vi "车牌识别模块.vi"(11 "图片路径":string="E:\\Program Files (x86)\\National Instruments\\LabVIEW 2013\\data\\记录照片\\00_20160426_110007.bmp") -> (0 "识别结果":T1, 3 "识别成功？":bool, 4 "加密狗插入？":bool)   [LabVIEW 2013]
uses:
  <vilib>/Utility/importsl/GetValueByPointer/datatype.ctl
  <vilib>/Utility/importsl/GetValueByPointer/GetValueByPointer.xnode
panel:
  out "pResult":string
  out "置信度":i32
  out "颜色":string
  out "车牌数目":i32
  out "左上Y":i32
  out "右下X":i32
  out "右下Y":i32
  out "左上X":i32
  out "车牌内容":string
  in  "HRIVLprOcx":refnum<k7>(container)
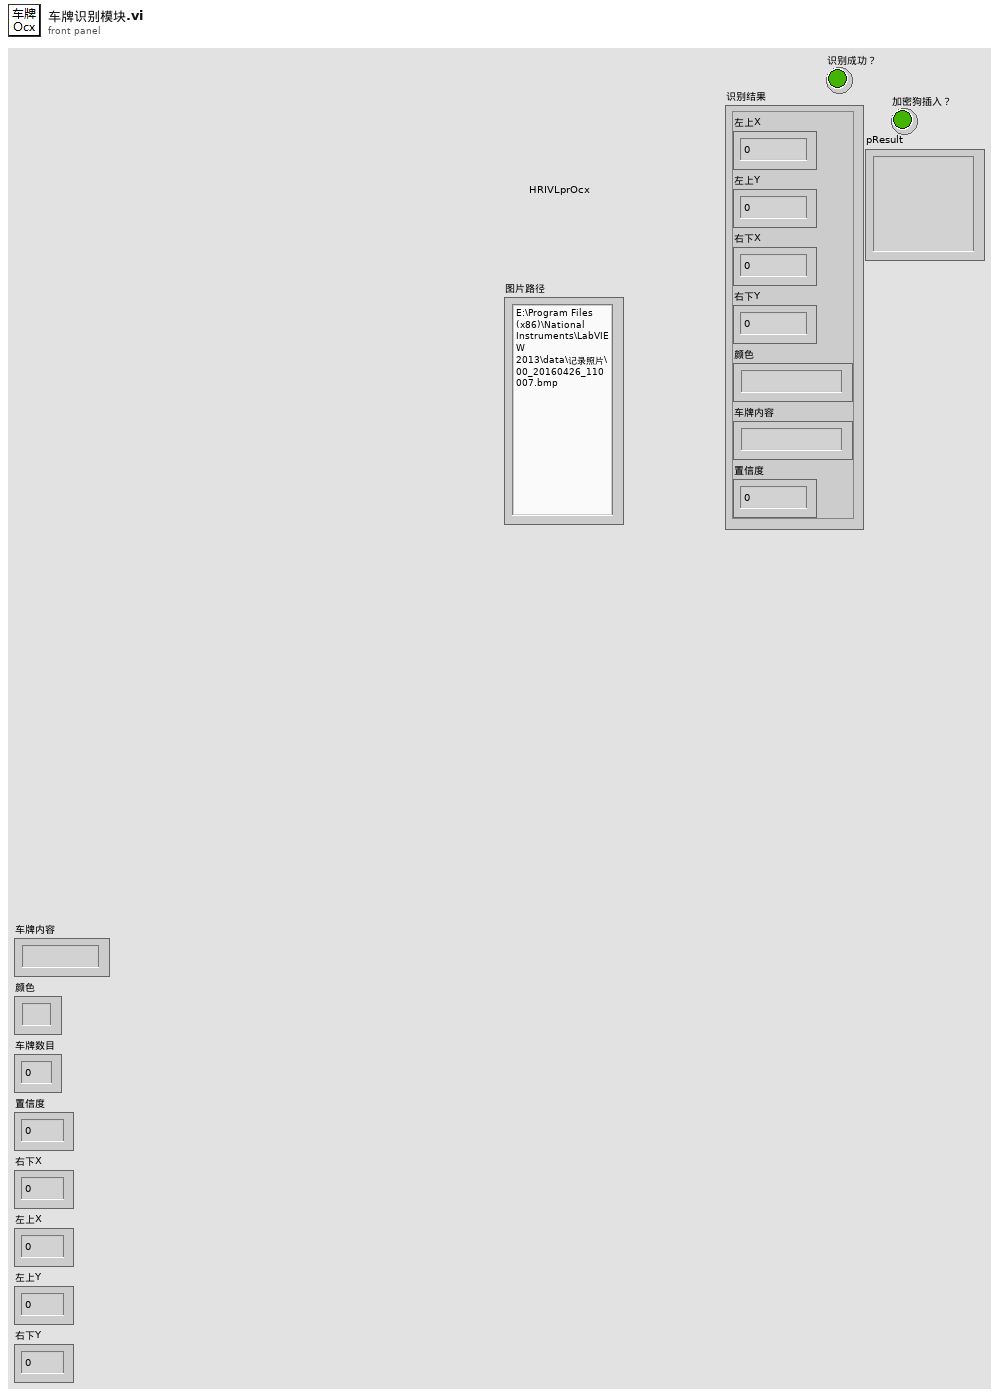
[diagram p1: front panel]
types:
  T1 = cluster{"左上X":i32, "左上Y":i32, "右下X":i32, "右下Y":i32, "颜色":string, "车牌内容":string, "置信度":i32}
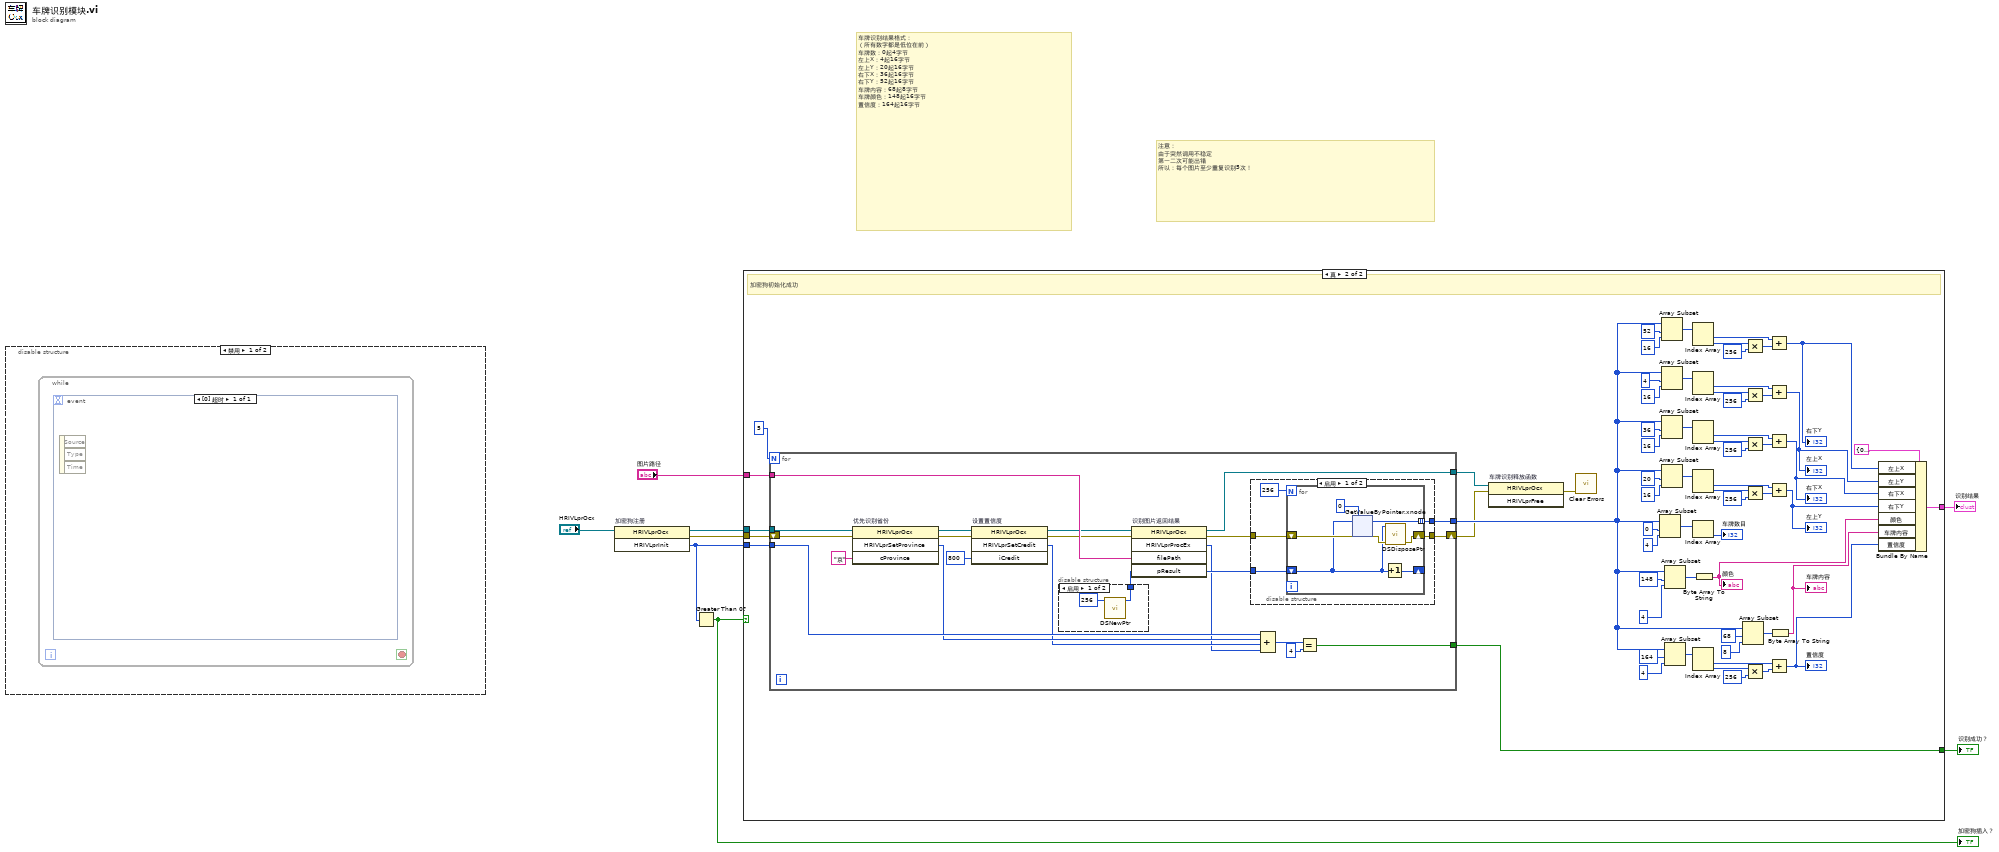
[diagram p0: block diagram]
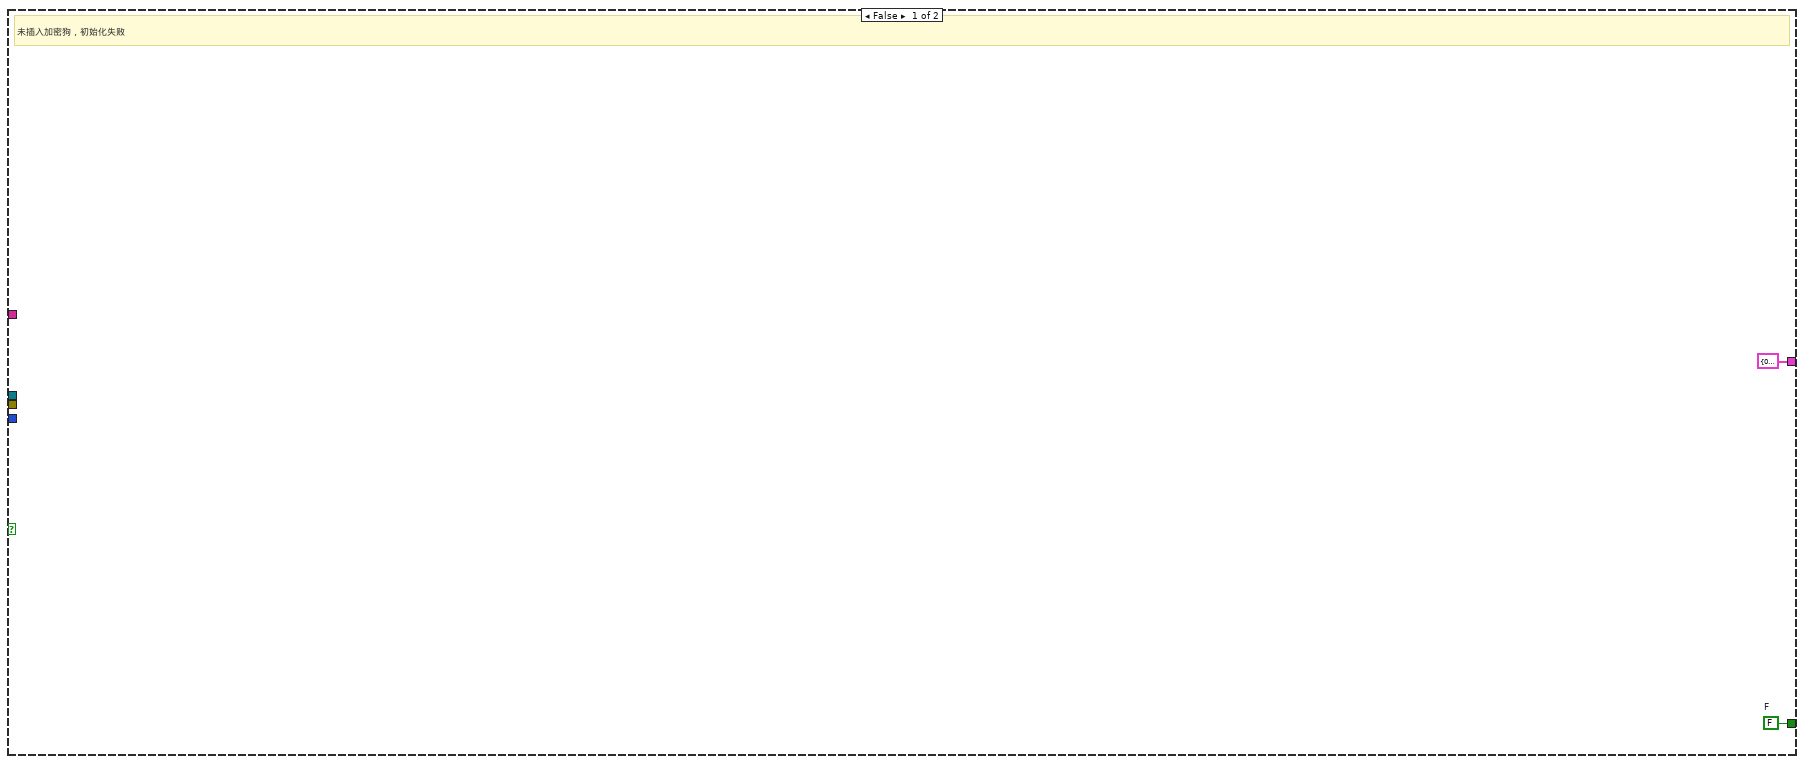
[diagram p3: hidden frame]
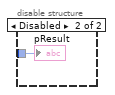
[diagram p5: hidden frame]
diagram:
  # "注意：\n由于突然调用不稳定\n第一二次可能出错\n所以：每个图片至少重复识别5次！"
  # "车牌识别结果格式：\n（所有数字都是低位在前）\n车牌数：0起4字节\n左上X：4起16字节\n左上Y：20起16字节\n右下X：36起16字节\n右下Y：52起16字节\n车牌内容：68起8字节\n车牌颜色：148起16字节\n置信度：164起16字节"
  n1 = disable-structure shown="禁用" {
    frame Disabled {
      n2 = while {
        stop <- _ stop-if-true
        n3 = event shown="[0] 超时" {
          selector: _ -> [_]
          dyn-events: _ -> [_]
          timeout: _ -> [_]
          event Timeout {
            n4 = event-data() -> ()  [unwired: 1 in, 3 out]
          }
        }
      }
    }
    frame Enabled {
    }
  }
  n5 = invoke on="加密狗注册" class="HRIVLprOcx" method="HRIVLprInit"(reference="HRIVLprOcx") -> (reference out=w7:refnum<k7>, error out=w4:errorcluster, "HRIVLprInit"=w1:i32)  [unwired: 2 in]
  n6 = Greater Than 0?(x=w1) -> (x > 0?=w2:bool)
  "加密狗插入？" <- w2
  n7 = case shown="真" w2 {
    tunnel: w7 -> [_ w74]
    tunnel: "图片路径" -> [_ w73]
    tunnel: w1 -> [_ w26]
    tunnel: [T1 {"左上X"=0, "左上Y"=0, "右下X"=0, "右下Y"=0, "颜色"="", "车牌内容"="", "置信度"=0} ("输出簇 2") w19] -> w5
    tunnel: w4 -> [_ w14]
    tunnel: [w10 w11] -> w3
    frame False {
      w10 = FALSE  # F
      # "未插入加密狗，初始化失败"
    }
    frame True {
      # "加密狗初始化成功"
      n8 = for {
        N: 5 -> [_]
        tunnel: w74 -> [w96]
        tunnel: w73 -> [w95]
        tunnel: [w94] -> w27
        tunnel: w26 -> [w93]
        tunnel: [w79] -> w15
        shift-right: [w78] -> w13
        shift-left: w14 -> [w77]
        tunnel: [w76] -> w11
        n9 = invoke on="优先识别省份" class="HRIVLprOcx" method="HRIVLprSetProvince"(reference=w96, error in=w77, "cProvince"="京") -> (reference out=w91:refnum<k7>, error out=w88:errorcluster, "HRIVLprSetProvince"=w85:i32)  [unwired: 1 in, 1 out]
        n10 = invoke on="设置置信度" class="HRIVLprOcx" method="HRIVLprSetCredit"(reference=w91, error in=w88, "iCredit"=800) -> (reference out=w89:refnum<k7>, error out=w87:errorcluster, "HRIVLprSetCredit"=w84:i32)  [unwired: 1 in, 1 out]
        n11 = disable-structure shown="启用" {
          disable-tunnel: [w97 _] -> w75
          frame Enabled {
            n12 = call <vilib>:"DSNewPtr.vi"("Size"=u64 256) -> ("Pointer"=w97:u64)  [unwired: 9 in, 1 out]
          }
          frame Disabled {
          }
        }
        n13 = invoke on="识别图片返回结果" class="HRIVLprOcx" method="HRIVLprProcEx"(reference=w89, error in=w87, "filePath"=w95, "pResult"=w75) -> (reference out=w79:refnum<k7>, error out=w80:errorcluster, "HRIVLprProcEx"=w83:i32, "pResult"=w86:i32)  [unwired: 1 in, 1 out]
        n14 = disable-structure shown="启用" {
          disable-tunnel: [w103 _] -> w94
          disable-tunnel: w86 -> [w101 w123]
          disable-tunnel: w80 -> [w100 _]
          disable-tunnel: [w99 _] -> w78
          frame Enabled {
            n15 = for {
              N: 256 -> [_]
              shift-right: [w110] -> _
              shift-left: w101 -> [w104]
              tunnel: [w108] -> w103 mode=indexing
              shift-right: [w105] -> w99
              shift-left: w100 -> [w107]
              n16 = xnode "GetValueByPointer.xnode"("Pointer"=w104, "InputType"=u8 0, "ErrorIn"=w107) -> ("Output"=w108:u8, "ErrorOut"=w106:errorcluster)  [unwired: 1 in]
              n17 = Increment(x=w104) -> (x+1=w110:i32)
              n18 = call <vilib>:"DSDisposePtr.vi"("error in (no error)"=w106, "Pointer"=w104) -> ("error out"=w105:errorcluster)  [unwired: 9 in]
            }
          }
          frame Disabled {
            "pResult" <- w123
          }
        }
        n19 = Compound Arithmetic op=ADD(w93, w85, w84, w83) -> (w82:i32)
        n20 = Equal?(x=w82, y=4) -> (x = y?=w76:bool)
      }
      n21 = invoke on="车牌识别释放函数" class="HRIVLprOcx" method="HRIVLprFree"(reference=w15, error in=w13) -> (error out=w12:errorcluster)  [unwired: 1 in, 2 out]
      n22 = call <vilib>:"Clear Errors.vi"("error in (no error)"=w12) -> ()  [unwired: 6 in, 1 out]
      n23 = Array Subset(array=w27, index=0 ("索引"), length=4 ("长度")) -> (w61:u8[])
      n24 = Array Subset(array=w27, index=52 ("索引"), length=16 ("长度")) -> (w60:u8[])
      n25 = Array Subset(array=w27, index=4 ("索引"), length=16 ("长度")) -> (w41:u8[])
      n26 = Array Subset(array=w27, index=36 ("索引"), length=16 ("长度")) -> (w59:u8[])
      n27 = Array Subset(array=w27, index=20 ("索引"), length=16 ("长度")) -> (w58:u8[])
      n28 = Array Subset(array=w27, index=148 ("索引"), length=4 ("长度")) -> (w65:u8[])
      n29 = Array Subset(array=w27, index=164 ("索引"), length=4 ("长度")) -> (w72:u8[])
      n30 = Index Array(array=w60) -> (element #1=w49:u8, element #2=w46:u8)  [unwired: 2 in]
      n31 = Index Array(array=w41) -> (element #1=w42:u8, element #2=w45:u8)  [unwired: 2 in]
      n32 = Index Array(array=w59) -> (element #1=w50:u8, element #2=w53:u8)  [unwired: 2 in]
      n33 = Index Array(array=w58) -> (element #1=w57:u8, element #2=w54:u8)  [unwired: 2 in]
      n34 = Index Array(array=w61) -> (element=→"车牌数目":u8)  [unwired: 1 in]
      n35 = Index Array(array=w72) -> (element #1=w68:u8, element #2=w71:u8)  [unwired: 2 in]
      n36 = Byte Array To String(unsigned byte array=w65) -> (string=w21:string)
      "颜色" <- w21
      n37 = Array Subset(array=w27, index=68 ("索引"), length=8 ("长度")) -> (w32:u8[])
      n38 = Multiply(x=w46, y=256) -> (x*y=w48:i32)
      n39 = Multiply(x=w45, y=256) -> (x*y=w43:i32)
      n40 = Multiply(x=w53, y=256) -> (x*y=w51:i32)
      n41 = Multiply(x=w54, y=256) -> (x*y=w56:i32)
      n42 = Multiply(x=w71, y=256) -> (x*y=w69:i32)
      n43 = Add(x=w49, y=w48) -> (x+y=w25:i32)
      "右下Y" <- w25
      n44 = Add(x=w42, y=w43) -> (x+y=w24:i32)
      "左上X" <- w24
      n45 = Add(x=w50, y=w51) -> (x+y=w23:i32)
      "右下X" <- w23
      n46 = Add(x=w57, y=w56) -> (x+y=w22:i32)
      "左上Y" <- w22
      n47 = Add(x=w68, y=w69) -> (x+y=w17:i32)
      "置信度" <- w17
      n48 = Byte Array To String(unsigned byte array=w32) -> (string=w20:string)
      "车牌内容" <- w20
      n49 = Bundle By Name(cluster=T1 {"左上X"=0, "左上Y"=0, "右下X"=0, "右下Y"=0, "颜色"="", "车牌内容"="", "置信度"=0} ("输出簇 2"), "左上X"=w25, "左上Y"=w24, "右下X"=w23, "右下Y"=w22, "颜色"=w21, "车牌内容"=w20, "置信度"=w17) -> (w19:T1)
    }
  }
  "识别结果" <- w5
  "识别成功？" <- w3
